vi "Clock.vi"(11 "Reset?":bool) -> (3 "Time Elapsed":dbl)   [LabVIEW 2014]
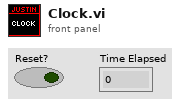
[diagram p1: front panel]
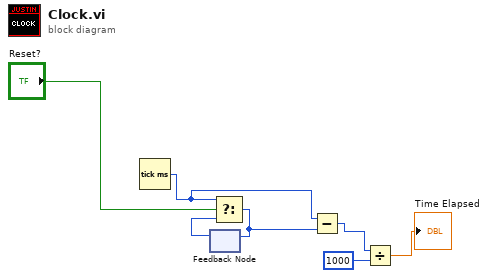
[diagram p0: block diagram]
diagram:
  n1 = Tick Count (ms)() -> (millisecond timer value=w2:u32)
  n2 = feedback #1() -> (w3:u32)  [unwired: 1 in]
  n3 = Select(t=w2, s="Reset?", f=w3) -> (s? t:f=w1:u32)
  n4 = feedback-in #1(w1) -> ()
  n5 = Subtract(x=w2, y=w1) -> (x-y=w5:u32)
  n6 = Divide(x=w5, y=u32 1000) -> (x/y=→"Time Elapsed":dbl)
